vi "SetpointFeedForward.vi"(7 "Reset":bool=TRUE, 8 "input valid":bool=TRUE, 9 "setpoint enabled":bool=TRUE, 10 "Samples to skip":u32=25, 11 "Data in":fxp<+/-,16,14>[](array[numeric])=[0.0, 0.0, 0.0, 0.0]) -> (0 "output valid":bool, 3 "Data out":fxp<+/-,16,14>[](array[numeric]))   [LabVIEW 2013]
doc: "Calculates various combinations on I_in, Q_in and cos(fi) and sin(fi) to be used later to delay the output signal"
uses:
  <vilib>/rvi/Memory/Memory_Emulation/niFpgaMemoryEmulationReadFromVariant.vi
  <vilib>/rvi/Emulation/niFpgaSctlEmulationGetInTimedLoop.vi
  <vilib>/rvi/Memory/Memory_Emulation/niFpgaMemoryEmulationWriteToVariant.vi
  <vilib>/rvi/DataTransferAndStorage/Container/Common/niFpgaContainerGetUniqueNameForEmu.vi
  <vilib>/rvi/errors/niFpgaSetErrorForExecOnDevCompSimple.vi
  <vilib>/rvi/Memory/Memory_Emulation/nirvimemoryFastEmulation.vi
  <vilib>/rvi/Memory/Memory_Emulation/nirvimemoryEmulation.vi
  <vilib>/rvi/DataTransferAndStorage/Container/XNode/niFpgaContainer.xnode
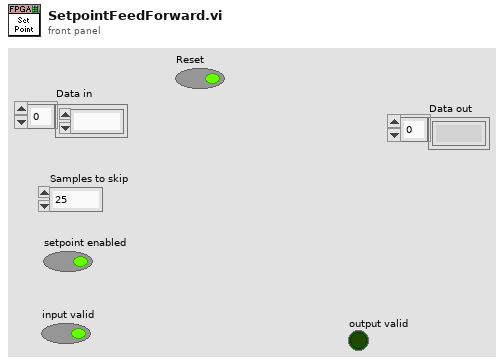
[diagram p1: front panel]
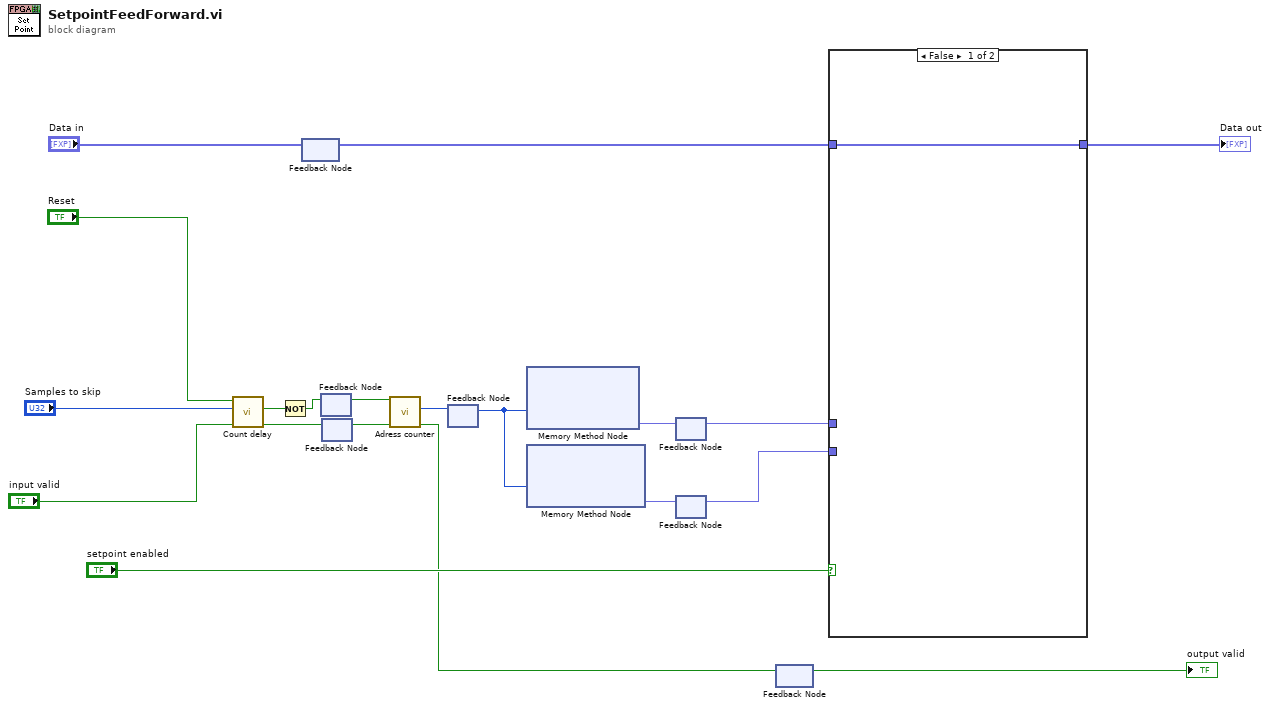
[diagram p0: block diagram]
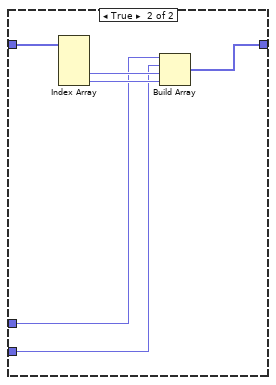
[diagram p2: hidden frame]
diagram:
  n1 = call "Count delay.vi"("input valid"="input valid", "Count to skip"="Samples to skip", "Reset"="Reset") -> ("output valid"=w16:bool, "count done?"=w17:bool)  [unwired: 7 in]
  n2 = Not(x=w17) -> (.not. x?=w13:bool)
  n3 = feedback #1() -> (w9:fxp<+/-,16,14>[])  [unwired: 1 in]
  n4 = feedback-in #1("Data in") -> ()
  n5 = feedback #2() -> (w14:bool)  [unwired: 1 in]
  n6 = feedback-in #2(w13) -> ()
  n7 = feedback-in #3(w16) -> ()
  n8 = feedback #3() -> (w15:bool)  [unwired: 1 in]
  n9 = call "Adress counter.vi"("input valid"=w15, "Reset"=w14) -> ("output valid"=w11:bool, "Address"=w2:u32)  [unwired: 8 in]
  n10 = feedback #4() -> (w1:u32)  [unwired: 1 in]
  n11 = feedback-in #4(w2) -> ()
  n12 = xnode ("Memory Method Node")("Address"=w1) -> ("Data"=w4:fxp<+/-,16,14>)  [unwired: 1 in, 1 out]
  n13 = xnode ("Memory Method Node")("Address"=w1) -> ("Data"=w3:fxp<+/-,16,14>)  [unwired: 1 in, 1 out]
  n14 = feedback #5() -> (w6:fxp<+/-,16,14>)  [unwired: 1 in]
  n15 = feedback-in #5(w4) -> ()
  n16 = feedback #6() -> (w5:fxp<+/-,16,14>)  [unwired: 1 in]
  n17 = feedback-in #6(w3) -> ()
  n18 = feedback #7() -> (→"output valid":bool)  [unwired: 1 in]
  n19 = feedback-in #7(w11) -> ()
  n20 = case shown="False" "setpoint enabled" {
    tunnel: w9 -> [w21 w27]
    tunnel: [w21 w24] -> w8
    tunnel: w6 -> [_ w22]
    tunnel: w5 -> [_ w23]
    frame False {
    }
    frame True {
      n21 = Index Array(array=w27) -> (element #3=w26:fxp<+/-,16,14>, element #4=w25:fxp<+/-,16,14>)  [unwired: 4 in, 2 out]
      n22 = Build Array(w22, w23, w26, w25) -> (w24:fxp<+/-,16,14>[])
    }
  }
  "Data out" <- w8
